vi "Distance.vi"(1 "B":cluster{"X":dbl, "Y":dbl}, 2 "A":cluster{"X":dbl, "Y":dbl}) -> (0 "Distance":dbl)   [LabVIEW 2015]
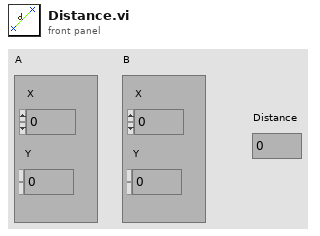
[diagram p1: front panel]
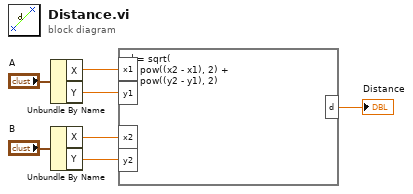
[diagram p0: block diagram]
diagram:
  n1 = Unbundle By Name("A") -> ("X"=w4:dbl, "Y"=w3:dbl)
  n2 = Unbundle By Name("B") -> ("X"=w2:dbl, "Y"=w1:dbl)
  n3 = formula code="d = sqrt(\n    pow((x2 - x1), 2) +\n    pow((y2 - y1), 2)\n);"("x1"=w4, "x2"=w2, "y1"=w3, "y2"=w1) -> ("d"=→"Distance":dbl)
